vi "AppClose.vi"(8 "Error In":errorcluster, 10 "This VI":refnum<vi>, 11 "This App":refnum<vi>) -> (0 "Error Out":errorcluster)   [LabVIEW 2017]
doc: "This SubVI check kind of current application. If it's in\nDevSys or other modes then do nothing. If it's in\nRun-Time mode then close FP of app."
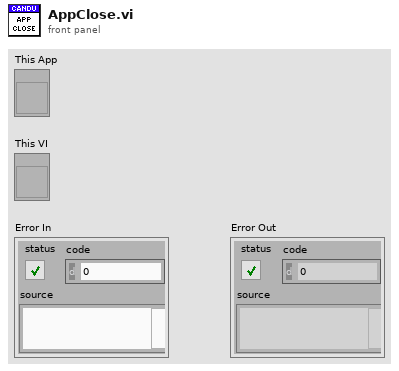
[diagram p1: front panel]
types:
  T1 = enum32{"invalid app kind", "Development System", "Run Time System", "Student Edition", "Embedded LabVIEW", "Evaluation", "Custom"}
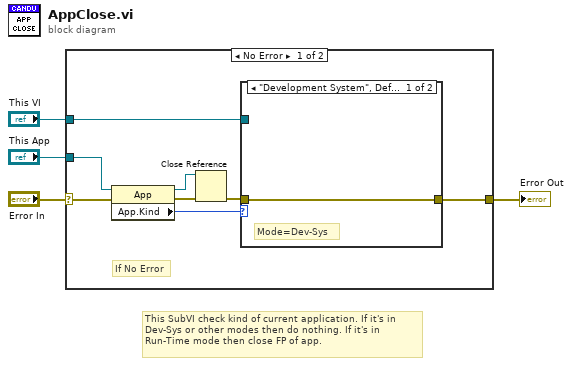
[diagram p0: block diagram]
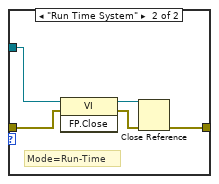
[diagram p2: hidden frame]
diagram:
  # "This SubVI check kind of current application. If it's in\nDev-Sys or other modes then do nothing. If it's in\nRun-Time mode then close FP of app."
  n1 = case shown="No Error" "Error In" {
    selector: "Error In" -> [w5 w19]
    tunnel: [w12 w19] -> w3
    tunnel: "This App" -> [w11 _]
    tunnel: "This VI" -> [w10 _]
    frame No Error {
      # "If No Error"
      n2 = property class="App"(reference=w11, error in=w5) -> (reference out=w6:refnum<vi>, error out=w8:errorcluster, "App.Kind"=w9:T1)
      n3 = Close Reference(reference=w6, error in (no error)=w8) -> (error out=w7:errorcluster)
      n4 = case shown="\"Development System\", Default" w9 {
        tunnel: w7 -> [w13 w16]
        tunnel: [w13 w15] -> w12
        tunnel: w10 -> [_ w14]
        frame "Development System", Default {
          # "Mode=Dev-Sys"
        }
        frame "Run Time System" {
          # "Mode=Run-Time"
          n5 = invoke class="VI" method="FP.Close"(reference=w14, error in=w16) -> (reference out=w18:refnum<vi>, error out=w17:errorcluster)  [unwired: 1 in, 1 out]
          n6 = Close Reference(reference=w18, error in (no error)=w17) -> (error out=w15:errorcluster)
        }
      }
    }
    frame Error {
      # "If any Error occurred"
    }
  }
  "Error Out" <- w3
